vi "RIO CAN Frame to Table on PC.vi"(5 "Widok ramek":bool, 7 "Hexadecimal?":bool, 9 "timestamp":timestamp, 10 "Input CAN Array":string[][](array[string]), 11 "CAN frame":T1 {"type" items=["CAN Data", "CAN Remote"]; "identifier" format="%.0x"}) -> (0 "ILE CAN FRAMES":dbl, 2 "string":string, 3 "Output CAN Array":string[][](array[string]), 4 "tekst":string, 6 "okres 100":dbl)   [LabVIEW 2015]
doc: "This example shows how to put a CAN transceiver to sleep on RIO Embedded CAN devices."
uses:
  CANFrameControl.ctl
panel:
  out "string 2":string
  out "substring before match":string
  out "subarray 2":string[](array[string])
  out "subarray":string[](array[string])
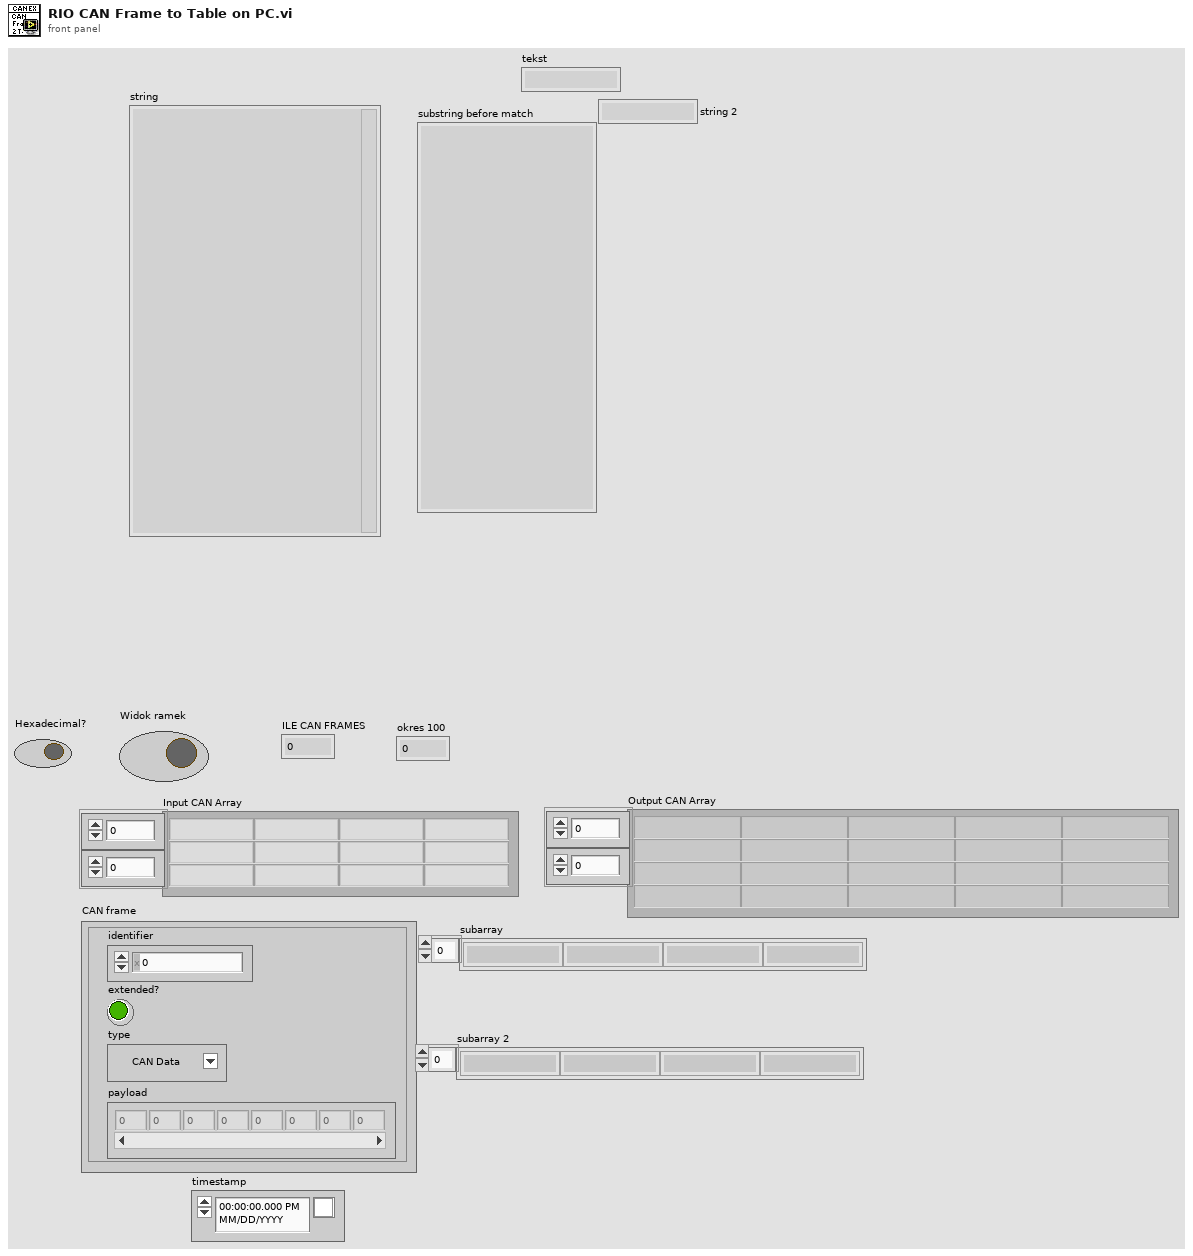
[diagram p1: front panel]
types:
  T1 = typedef "CANFrameControl.ctl" = cluster{"identifier":u32, "extended?":bool, "type":u8, "payload":u8[]}
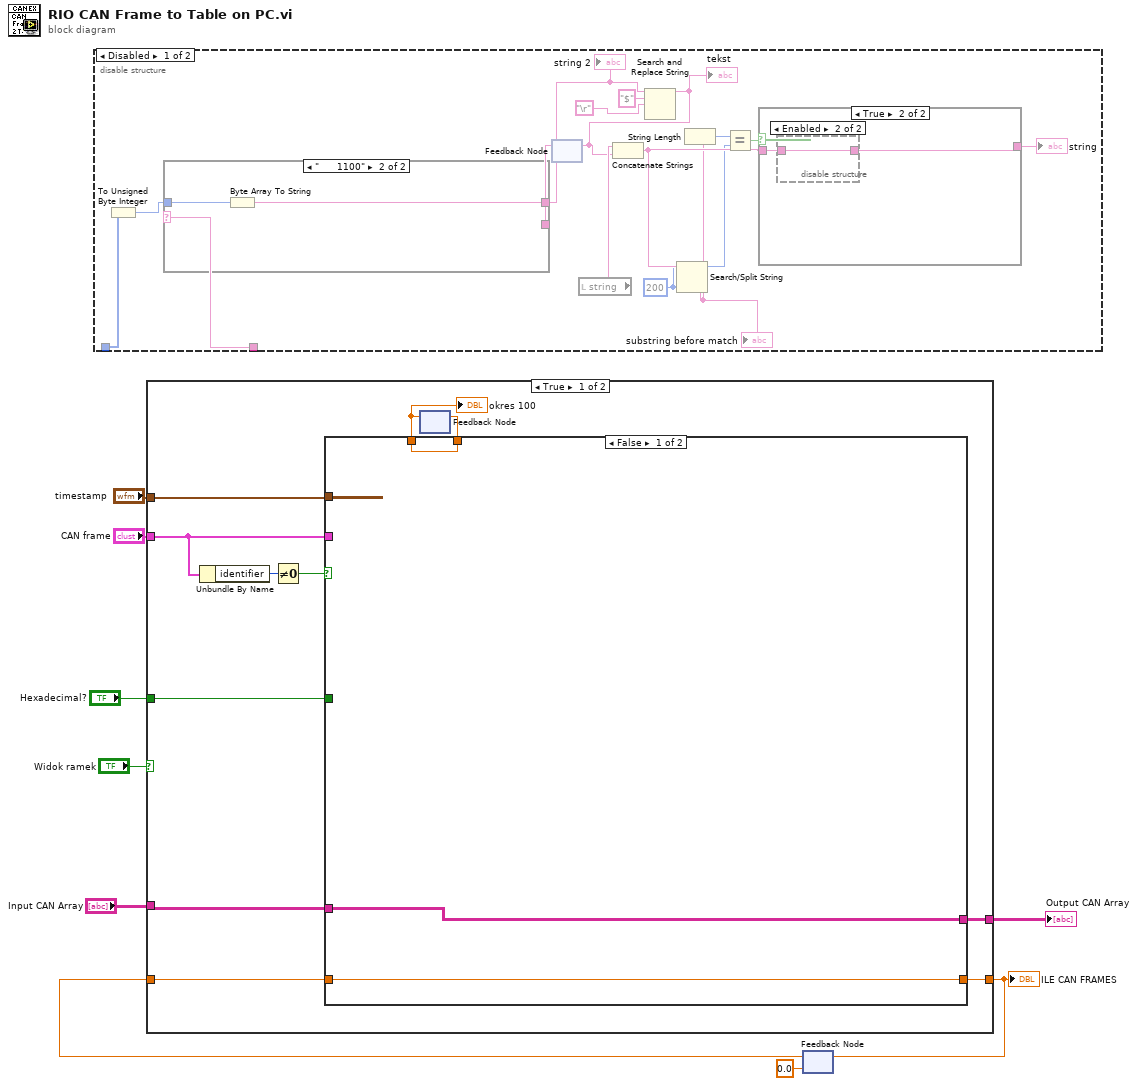
[diagram p0: block diagram]
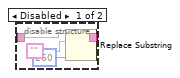
[diagram p3: hidden frame]
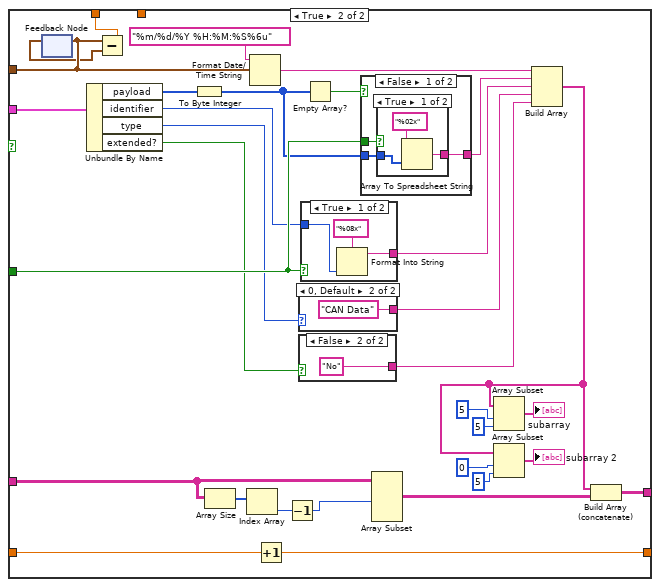
[diagram p6: hidden frame]
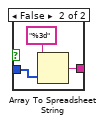
[diagram p7: hidden frame]
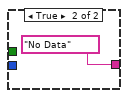
[diagram p8: hidden frame]
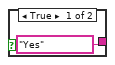
[diagram p9: hidden frame]
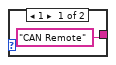
[diagram p10: hidden frame]
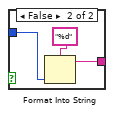
[diagram p11: hidden frame]
diagram:
  n1 = disable-structure shown="Disabled" {
    disable-tunnel: _ -> [w24 _]
    disable-tunnel: _ -> [w10 _]
    frame Disabled {
      w12 = 200 ("offset (0)")
      n2 = To Unsigned Byte Integer(number=w10) -> (unsigned 8bit integer=w11:u8)
      n3 = feedback #1() -> (w23:string)  [unwired: 1 in]
      n4 = case shown="\"      1100\"" w24 {
        tunnel: w11 -> [_ w35]
        tunnel: [w33 w34] -> w20
        tunnel: w23 -> [w33 _]
        frame "False", Default {
        }
        frame "      1100" {
          n5 = Byte Array To String(unsigned byte array=w35) -> (string=w34:string)
        }
      }
      "string 2" <- w20
      n6 = local read "string"() -> (w18:string)
      n7 = Search and Replace String(input string=w20, search string="$", replace string="\r") -> (result string=w16:string)  [unwired: 5 in, 3 out]
      "tekst" <- w16
      n8 = feedback-in #1(w16) -> ()
      n9 = Concatenate Strings(w18, w16) -> (w17:string)
      n10 = Search/Split String(string=w17, offset (0)=w12) -> (substring before match=w13:string)  [unwired: 1 in, 2 out]
      "substring before match" <- w13
      n11 = String Length(string=w13) -> (length=w15:i32)
      n12 = Equal?(x=w15, y=w12) -> (x = y?=w14:bool)
      n13 = case shown="True" w14 {
        tunnel: [w25 w27] -> w19
        tunnel: w17 -> [w25 w26]
        frame False {
        }
        frame True {
          n14 = disable-structure shown="Enabled" {
            disable-tunnel: [w31 w32] -> w27
            disable-tunnel: w26 -> [w30 w32]
            frame Disabled {
              n15 = Replace Substring(2:260 ("length (len. of substring)"), 4:"", 5:w30) -> (1:w31:string)  [unwired: 1 in, 1 out]
            }
            frame Enabled {
            }
          }
        }
      }
      "string" <- w19
    }
    frame Enabled {
    }
  }
  n16 = feedback #2(0.0) -> (w3:dbl)
  n17 = case shown="True" "Widok ramek" {
    tunnel: "Input CAN Array" -> [w44 w103]
    tunnel: [w46 w103] -> w6
    tunnel: "Hexadecimal?" -> [w45 _]
    tunnel: "CAN frame" -> [w41 _]
    tunnel: "timestamp" -> [w39 _]
    tunnel: [w43 w102] -> w2
    tunnel: w3 -> [w42 w102]
    frame True {
      n18 = Unbundle By Name(w41) -> ("identifier"=w38:u32)
      n19 = Not Equal To 0?(x=w38) -> (x != 0?=w40:bool)
      n20 = feedback #3() -> (w36:dbl)  [unwired: 1 in]
      n21 = case shown="False" w40 {
        tunnel: [w48 w81] -> w46
        tunnel: w45 -> [_ w80]
        tunnel: w39 -> [_ w52]
        tunnel: w44 -> [w48 w79]
        tunnel: w41 -> [_ w78]
        tunnel: [w49 w77] -> w43
        tunnel: w42 -> [w49 w76]
        tunnel: [w47 w50] -> w37
        tunnel: w36 -> [w47 _]
        frame False {
        }
        frame True {
          n22 = feedback #4() -> (w51:timestamp)  [unwired: 1 in]
          n23 = feedback-in #4(w52) -> ()
          n24 = Unbundle By Name(w78) -> ("payload"=w54:u8[], "identifier"=w56:u32, "type"=w65:u8, "extended?"=w62:bool)
          n25 = Subtract(x=w52, y=w51) -> (x-y=w50:dbl)
          n26 = To Byte Integer(number=w54) -> (8bit integer=w53:i8[])
          n27 = Array Size(array=w79) -> (size(s)=w75:i32[])
          n28 = Index Array(array=w75) -> (element=w74:i32)  [unwired: 1 in]
          n29 = Format Date/Time String(time format string (%c)="%m/%d/%Y %H:%M:%S%6u", seconds (now)=w52) -> (date/time string=w66:string)  [unwired: 1 in]
          n30 = Increment(x=w76) -> (x+1=w77:dbl)
          n31 = Decrement(x=w74) -> (x-1=w57:i32)
          n32 = case shown="0, Default" w65 {
            tunnel: ["CAN Remote" "CAN Data"] -> w64
            frame 1 {
            }
            frame 0, Default {
            }
          }
          n33 = case shown="False" w62 {
            tunnel: ["Yes" "No"] -> w63
            frame True {
            }
            frame False {
            }
          }
          n34 = case shown="True" w80 {
            tunnel: w56 -> [w97 w100]
            tunnel: [w96 w99] -> w55
            frame True {
              n35 = Format Into String(format string="%08x", w97) -> (resulting string=w96:string)  [unwired: 2 in, 1 out]
            }
            frame False {
              n36 = Format Into String(format string="%d", w100) -> (resulting string=w99:string)  [unwired: 2 in, 1 out]
            }
          }
          n37 = Empty Array?(array=w53) -> (empty?=w59:bool)
          n38 = case shown="False" w59 {
            tunnel: [w83 "No Data"] -> w61
            tunnel: w53 -> [w82 _]
            tunnel: w80 -> [w84 _]
            frame False {
              n39 = case shown="True" w84 {
                tunnel: w82 -> [w85 w88]
                tunnel: [w86 w89] -> w83
                frame True {
                  n40 = Array To Spreadsheet String(array=w85, 3:"%02x" ("format string")) -> (spreadsheet string=w86:string)  [unwired: 1 in]
                }
                frame False {
                  n41 = Array To Spreadsheet String(array=w88, 3:"%3d" ("format string")) -> (spreadsheet string=w89:string)  [unwired: 1 in]
                }
              }
            }
            frame True {
            }
          }
          n42 = Array Subset(array=w79, length (row)=w57) -> (w67:string[][])  [unwired: 3 in]
          n43 = Build Array(w66, w61, w55, w64, w63) -> (w58:string[])
          n44 = Array Subset(array=w58, index=5 ("length"), length=5) -> (→"subarray":string[])
          n45 = Array Subset(array=w58, index=0 ("length"), length=5) -> (→"subarray 2":string[])
          n46 = Build Array (concatenate)(w58, w67) -> (w81:string[][])
        }
      }
      "okres 100" <- w37
      n47 = feedback-in #3(w37) -> ()
    }
    frame False {
    }
  }
  "Output CAN Array" <- w6
  "ILE CAN FRAMES" <- w2
  n48 = feedback-in #2(w2) -> ()
